vi "Move Selection.vi"(5 "Waveform Graph":T1, 7 "Timeline":T5, 8 "error in (no error)":errorcluster, 9 "Coords":T2, 11 "Xinformation In":T3) -> (0 "error out":errorcluster, 3 "Xinformation Out":T3)   [LabVIEW 2013, in "XGrapher.xctl"]
doc: "This vi handles when the user has grabbed the timline and dragged to the left and right. This also prevents the user from dragging too far to the right or the left (outside the timeline span)"
uses:
  XGrapher.xctl
  Typedefs/Xctrl-Timeline graph ref.ctl
  Typedefs/Xinformation.ctl
  Typedefs/Xcrtl-Click Operation.ctl
  <vilib>/Utility/miscctls.llb/LVPoint32TypeDef.ctl
  Typedefs/Xctrl-Waveform graph ref.ctl
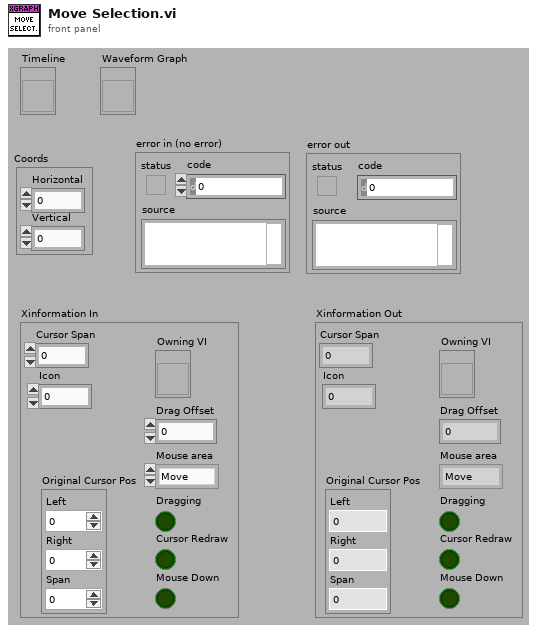
[diagram p1: front panel]
types:
  T1 = typedef "XGrapher.xctl/Xctrl-Waveform graph ref.ctl" = refnum<vi>
  T2 = typedef "LVPoint32TypeDef.ctl" = cluster{"Horizontal":i32, "Vertical":i32}
  T3 = typedef "XGrapher.xctl/Xinformation.ctl" = cluster{"Cursor Span":dbl, "Icon":u16, "Mouse Down":bool, "Owning VI":refnum<vi>, "Mouse area":T4, "Dragging":bool, "Drag Offset":dbl, "Original Cursor Pos":cluster{"Left":dbl, "Right":dbl, "Span":dbl}, "Cursor Redraw":bool}
  T4 = typedef "XGrapher.xctl/Xcrtl-Click Operation.ctl" = enum16{"Move", "left cursor", "right cursor", "none"}
  T5 = typedef "XGrapher.xctl/Xctrl-Timeline graph ref.ctl" = refnum<vi>
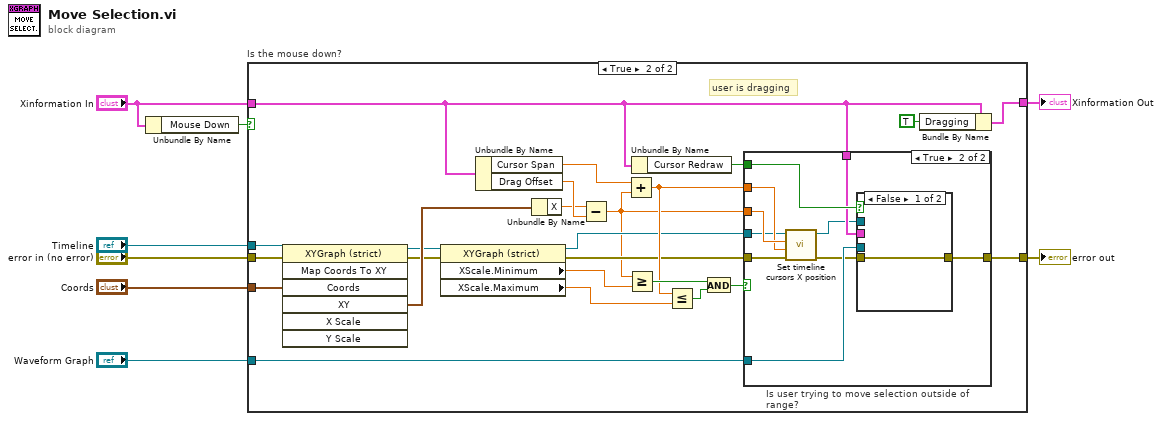
[diagram p0: block diagram]
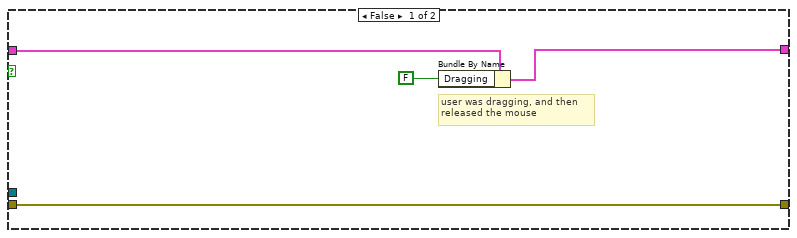
[diagram p2: hidden frame]
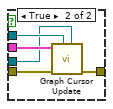
[diagram p4: hidden frame]
diagram:
  n1 = Unbundle By Name("Xinformation In") -> ("Mouse Down"=w7:bool)
  n2 = case "Is the mouse down?" shown="True" w7 {
    tunnel: "Coords" -> [_ w26]
    tunnel: "Xinformation In" -> [w11 w15]
    tunnel: [w10 w34] -> w6
    tunnel: "Timeline" -> [_ w24]
    tunnel: "error in (no error)" -> [w9 w23]
    tunnel: [w9 w20] -> w2
    tunnel: "Waveform Graph" -> [_ w19]
    frame False {
      # "user was dragging, and then \nreleased the mouse"
      n3 = Bundle By Name(cluster=w11, "Dragging"=FALSE) -> (w10:T3)
    }
    frame True {
      # "user is dragging"
      n4 = invoke on="Invoke Node" class="XYGraph (strict)" method="Map Coords To XY"(reference=w24, error in=w23, "Coords"=w26) -> (reference out=w18:T5, error out=w22:errorcluster, "XY"=w36:cluster{"X":dbl, "Y":dbl})  [unwired: 4 in, 4 out]
      n5 = property on="Property Node" class="XYGraph (strict)"(reference=w18, error in=w22) -> (reference out=w17:T5, error out=w21:errorcluster, "XScale.Minimum"=w32:dbl, "XScale.Maximum"=w29:dbl)
      n6 = Unbundle By Name(w15) -> ("Cursor Span"=w13:dbl, "Drag Offset"=w35:dbl)
      n7 = Unbundle By Name(w36) -> ("X"=w25:dbl)
      n8 = Subtract(x=w25, y=w35) -> (x-y=w14:dbl)
      n9 = Add(x=w13, y=w14) -> (x+y=w30:dbl)
      n10 = Greater Or Equal?(x=w14, y=w32) -> (x >= y?=w31:bool)
      n11 = Unbundle By Name(w15) -> ("Cursor Redraw"=w16:bool)
      n12 = Less Or Equal?(x=w30, y=w29) -> (x <= y?=w28:bool)
      n13 = And(x=w31, y=w28) -> (x .and. y?=w27:bool)
      n14 = case "Is user trying to move selection outside of range?" shown="True" w27 {
        tunnel: w30 -> [_ w42]
        tunnel: w14 -> [_ w43]
        tunnel: w19 -> [_ w47]
        tunnel: w17 -> [_ w41]
        tunnel: w21 -> [w37 w38]
        tunnel: [w37 w46] -> w20
        tunnel: w16 -> [_ w45]
        tunnel: w15 -> [_ w44]
        frame False {
          # "Move is occuring outside of \ntimeline range, ignore drag request"
        }
        frame True {
          n15 = call "Set timeline cursors X position.vi"("error in (no error)"=w38, "Right"=w42, "Left"=w43, "Timeline Graph in"=w41) -> ("error out"=w39:errorcluster, "Timeline Graph out"=w40:T5)  [unwired: 6 in]
          n16 = case shown="False" w45 {
            tunnel: w47 -> [_ w49]
            tunnel: w44 -> [_ w53]
            tunnel: w40 -> [_ w52]
            tunnel: w39 -> [w48 w51]
            tunnel: [w48 w50] -> w46
            frame False {
            }
            frame True {
              n17 = call "Graph Cursor Update.vi"("Waveform Ref in"=w49, "Timeline Ref in"=w52, "error in (no error)"=w51, "Xinformation In"=w53) -> ("error out"=w50:errorcluster)  [unwired: 5 in, 2 out]
            }
          }
        }
      }
      n18 = Bundle By Name(cluster=w15, "Dragging"=TRUE) -> (w34:T3)
    }
  }
  "Xinformation Out" <- w6
  "error out" <- w2
